vi "ScaledWaveform-GetChannelRefs.vi"(8 "Error in":errorcluster, 9 "Enabled?":bool, 11 "Device Ref in":T1 format="%.0x") -> (0 "Error out":errorcluster, 2 "Channel Refs Array":T1[](array[typedef]) format="%.0x", 3 "Device Ref out":T1=18446744073709551615 format="%.0x")   [LabVIEW 2015, in "Waveform-Processing-Custom-Device Shared.lvlib" / "Scaled Waveform.lvlib"]
uses:
  Scaled Waveform.lvlib
  <vilib>/NI Veristand/Custom Device API/Custom Device Item Ref.ctl
  Constants.vi
  <vilib>/NI Veristand/Custom Device API/Get Item Property (Dependent Node Pointer).vi
  System Explorer/Waveform-Processing-Custom-Device System Explorer.lvlib
  <vilib>/NI VeriStand/Custom Device API/Custom Device API.lvlib
  Waveform-Processing-Custom-Device Shared.lvlib
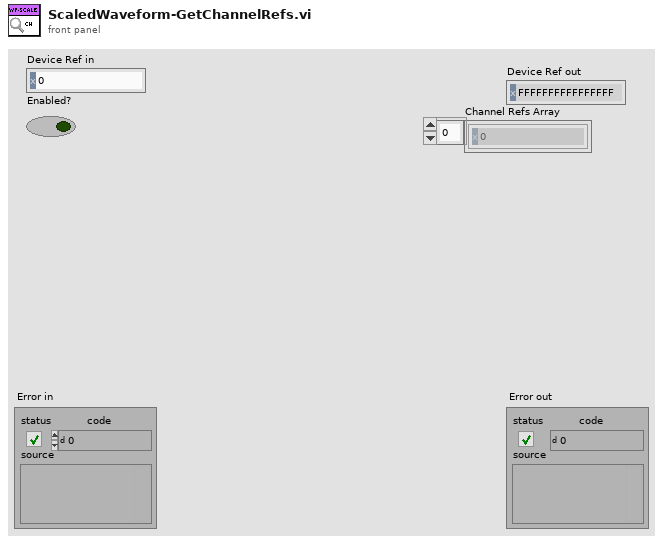
[diagram p1: front panel]
types:
  T1 = typedef "Custom Device API.lvlib/Custom Device Item Ref.ctl" = u64
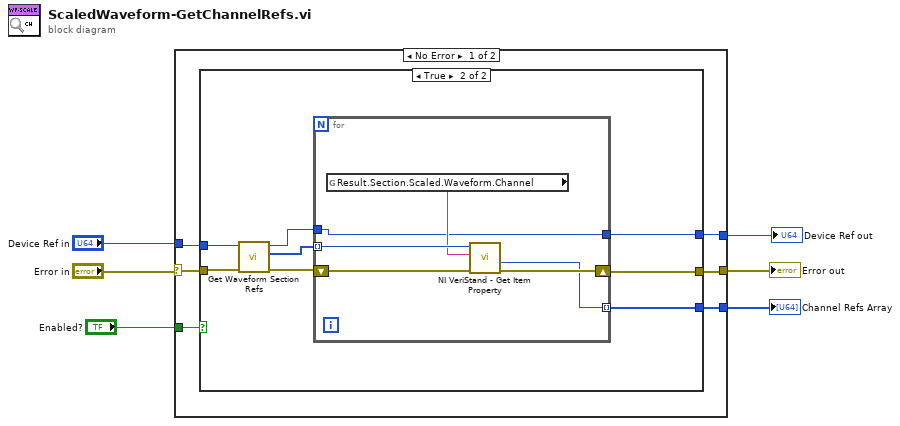
[diagram p0: block diagram]
diagram:
  n1 = case shown="No Error" "Error in" {
    selector: "Error in" -> [w12 w30]
    tunnel: [w10 w30] -> w3
    tunnel: "Device Ref in" -> [w11 w29]
    tunnel: "Enabled?" -> [w9 _]
    tunnel: [w8 w29] -> w6
    tunnel: [w7 _] -> w1
    frame No Error {
      n2 = case shown="True" w9 {
        tunnel: w12 -> [w14 w22]
        tunnel: w11 -> [w13 w21]
        tunnel: [w14 w17] -> w10
        tunnel: [w13 w16] -> w8
        tunnel: [_ w15] -> w7
        frame False {
        }
        frame True {
          n3 = call "Get Waveform Section Refs.vi"("Error in"=w22, "Device Ref in"=w21) -> ("Error out"=w20:errorcluster, "Result Section Refs"=w19:T1[], "Device Ref out"=w18:T1)  [unwired: 7 in]
          n4 = for {
            tunnel: w19 -> [w27] mode=indexing
            tunnel: w18 -> [w23]
            shift-right: [w25] -> w17
            shift-left: w20 -> [w28]
            tunnel: [w24] -> w15 mode=indexing
            tunnel: [w23] -> w16
            n5 = global read "Constants.vi" "Result.Section.Scaled.Waveform.Channel"() -> (w26:string)
            n6 = call-poly <vilib>:"NI VeriStand - Get Item Property.vi"("error in (no error)"=w28, "Property Name"=w26, "Item Ref in"=w27) -> ("error out"=w25:errorcluster, "Dependent Node Ref"=w24:T1)  [unwired: 5 in, 2 out]
          }
        }
      }
    }
    frame Error {
    }
  }
  "Error out" <- w3
  "Device Ref out" <- w6
  "Channel Refs Array" <- w1
